vi "ps_read.vi"(8 "error in (no error)":errorcluster, 11 "Instrument in":refnum<class "Instrument.lvclass">) -> (0 "error out":errorcluster, 1 "OutputCurrent":sgl, 2 "OutputVoltage":sgl, 3 "Instrument out":refnum<class "Instrument.lvclass">, 4 "AlertCode":i8, 5 "isStopped":bool, 6 "EmergencyState":i8)   [LabVIEW 2019, in "Instrument.lvclass"]
uses:
  Instrument.lvclass
  Instrument.lvclass/Instrument.ctl
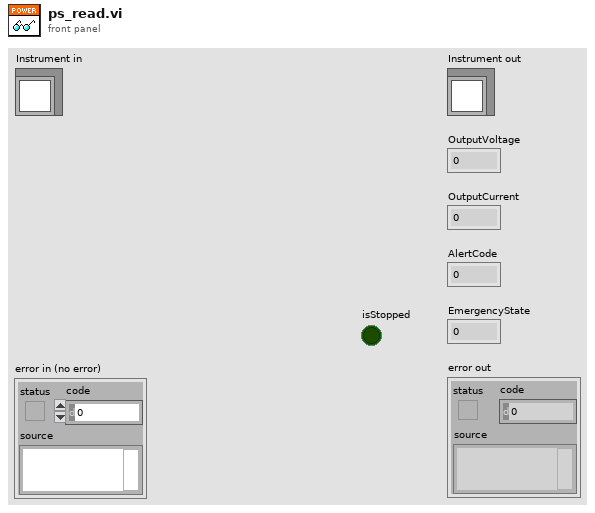
[diagram p1: front panel]
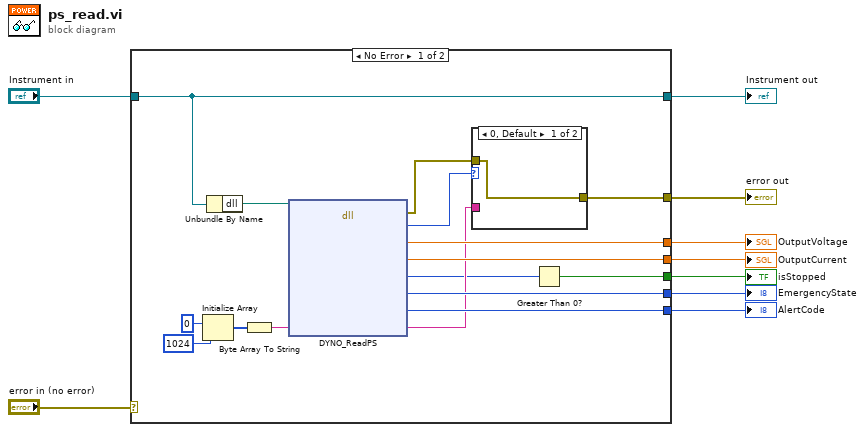
[diagram p0: block diagram]
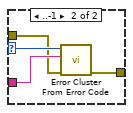
[diagram p2: hidden frame]
diagram:
  n1 = case shown="No Error" "error in (no error)" {
    selector: "error in (no error)" -> [_ w32]
    tunnel: [w12 w32] -> w8
    tunnel: [w25 w31] -> w6
    tunnel: "Instrument in" -> [w25 w31]
    tunnel: [w23 _] -> w5
    tunnel: [w22 _] -> w4
    tunnel: [w21 _] -> w3
    tunnel: [w20 _] -> w2
    tunnel: [w10 _] -> w1
    frame No Error {
      n2 = Initialize Array(u8 0 ("element"), 1024 ("dimension size")) -> (w17:u8[])
      n3 = Unbundle By Name(w25) -> ("dll"=w24:path)
      n4 = Byte Array To String(unsigned byte array=w17) -> (string=w16:string)
      n5 = dll-call lib="C:/Dev/22KW-Dyno/software/data/DynoAPI.dll" fn="DYNO_ReadPS"(path in=w24, "ErrorMsg"=w16) -> (error out=w14:errorcluster, "return type"=w15:i32, "OutputVoltage"=w23:sgl, "OutputCurrent"=w22:sgl, "IsStopped"=w11:i8, "EmergencyState"=w21:i8, "AlertCode"=w20:i8, "ErrorMsg"=w13:string)  [unwired: 7 in, 1 out]
      n6 = case shown="0, Default" w15 {
        selector: w15 -> [_ w30]
        tunnel: w13 -> [_ w29]
        tunnel: w14 -> [w26 w28]
        tunnel: [w26 w27] -> w12
        frame 0, Default {
        }
        frame ..-1 {
          n7 = call <vilib>:"Error Cluster From Error Code.vi"("error in (no error)"=w28, "error message (\"\")"=w29, "error code (0)"=w30) -> ("error out"=w27:errorcluster)  [unwired: 6 in]
        }
      }
      n8 = Greater Than 0?(x=w11) -> (x > 0?=w10:bool)
    }
    frame Error {
    }
  }
  "error out" <- w8
  "Instrument out" <- w6
  "OutputVoltage" <- w5
  "OutputCurrent" <- w4
  "isStopped" <- w1
  "EmergencyState" <- w3
  "AlertCode" <- w2
